vi "SrvGetParam.vi"(0 "ref in":u64, 7 "ParamNumber":i32(ring)=131 items=["Local Port"=1, "Remote Port"=2, "Ping Timeout (ms)"=3, "Send Timeout (ms)"=4, "Recv Timeout (ms)"=5, "Work Interval (ms)"=6, "Source REF"=7, "Destination REF"=8, "Source TSAP"=9, "PDU Request"=10, "Max Clients"=11, "BSend Timeout (ms)"=12, "BRecv Timeout (ms)"=13, "Recovery Time (ms)"=14, "Keep Alive Time (ms)"=15], 11 "error in (no error)":errorcluster) -> (4 "ref out":u64, 6 "Result":i32, 8 "ParamValue":i32, 15 "error out":errorcluster)   [LabVIEW 2010, in "Snap7.lvlib"]
uses:
  Snap7.lvlib
  windows/lv_snap7.dll
panel:
  in  "U32":u32
  in  "U16":u16
  in  "I32":i32
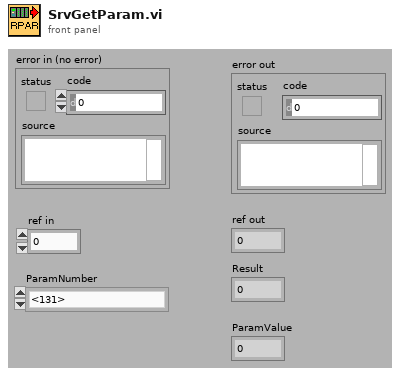
[diagram p1: front panel]
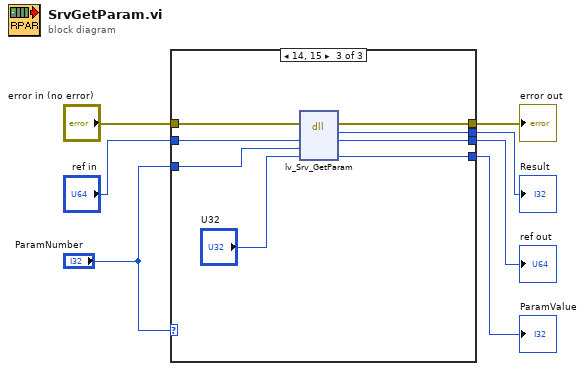
[diagram p0: block diagram]
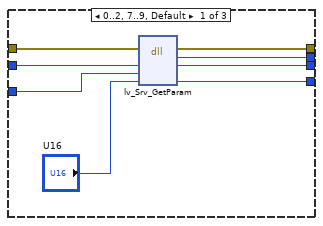
[diagram p2: hidden frame]
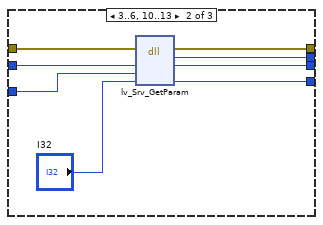
[diagram p3: hidden frame]
diagram:
  n1 = case shown="14, 15" "ParamNumber" {
    tunnel: "ref in" -> [w13 w23 w29]
    tunnel: [w10 w22 w26] -> w6
    tunnel: [w9 w21 w25] -> w5
    tunnel: "error in (no error)" -> [w14 w20 w30]
    tunnel: [w11 w19 w27] -> w3
    tunnel: [w8 w18 w24] -> w2
    tunnel: "ParamNumber" -> [w12 w17 w28]
    frame 0..2, 7..9, Default {
      n2 = dll-call lib="C:/snap7-src-1.0.0/LabVIEW/lib/windows/lv_snap7.dll" fn="lv_Srv_GetParam"(error in=w14, "Client"=w13, "ParamNumber"=w12, "ParamValue"="U16") -> (error out=w11:errorcluster, "return type"=w10:i32, "Client"=w9:u64, "ParamValue"=w8:u16)  [unwired: 3 in, 1 out]
    }
    frame 3..6, 10..13 {
      n3 = dll-call lib="C:/snap7-src-1.0.0/LabVIEW/lib/windows/lv_snap7.dll" fn="lv_Srv_GetParam"(error in=w20, "Client"=w23, "ParamNumber"=w17, "ParamValue"="I32") -> (error out=w19:errorcluster, "return type"=w22:i32, "Client"=w21:u64, "ParamValue"=w18:i32)  [unwired: 3 in, 1 out]
    }
    frame 14, 15 {
      n4 = dll-call lib="C:/snap7-src-1.0.0/LabVIEW/lib/windows/lv_snap7.dll" fn="lv_Srv_GetParam"(error in=w30, "Client"=w29, "ParamNumber"=w28, "ParamValue"="U32") -> (error out=w27:errorcluster, "return type"=w26:i32, "Client"=w25:u64, "ParamValue"=w24:u32)  [unwired: 3 in, 1 out]
    }
  }
  "Result" <- w6
  "ref out" <- w5
  "error out" <- w3
  "ParamValue" <- w2
